vi "WFT I2C Configure Port.vi"(8 "Error In":errorcluster, 9 "SDA idxChannel":i32=1, 10 "SCL idxChannel":i32, 11 "WaveForms Session In":T1) -> (0 "Error Out":errorcluster, 1 "ret_sda":i32, 2 "ret_scl":i32, 3 "WaveForms Session Out":T1)   [LabVIEW 2020, in "lv_waveforms_toolkit.lvlib"]
uses:
  lv_waveforms_toolkit.lvlib
  WFT Session.ctl
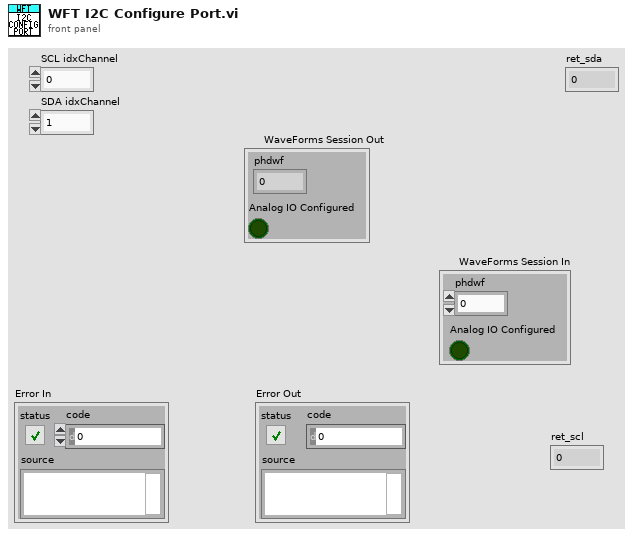
[diagram p1: front panel]
types:
  T1 = typedef "lv_waveforms_toolkit.lvlib/WFT Session.ctl" = cluster{"phdwf":i32, "Analog IO Configured":bool}
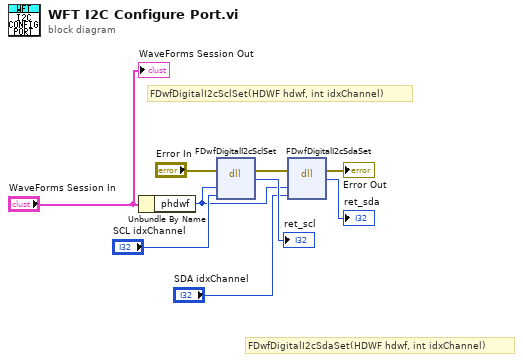
[diagram p0: block diagram]
diagram:
  # "FDwfDigitalI2cSdaSet(HDWF hdwf, int idxChannel)"
  # "FDwfDigitalI2cSclSet(HDWF hdwf, int idxChannel)"
  n1 = Unbundle By Name("WaveForms Session In") -> ("phdwf"=w2:i32)
  n2 = dll-call lib="dwf" fn="FDwfDigitalI2cSclSet"(error in="Error In", "phdwf"=w2, "idxChannel"="SCL idxChannel") -> (error out=w5:errorcluster, "return type"=→"ret_scl":i32)  [unwired: 4 in, 1 out]
  n3 = dll-call lib="dwf" fn="FDwfDigitalI2cSdaSet"(error in=w5, "phdwf"=w2, "idxChannel"="SDA idxChannel") -> (error out=→"Error Out":errorcluster, "return type"=→"ret_sda":i32)  [unwired: 4 in, 1 out]
  "WaveForms Session Out" <- "WaveForms Session In"
